vi "车牌字母识别.vi"() -> ()   [LabVIEW 2020]
uses:
  <vilib>/userdefined/High Color/IMAQdx.ctl
  <vilib>/vision/driver/NI_Vision_Acquisition_Software.lvlib
  <vilib>/vision/NI_Vision_Development_Module.lvlib
panel:
  out "Read String":string
  in  "停止":bool
  out "Image":T1(plugin-control)
  in  "Rectangle":T2 {"Rotation" min=-90.0 max=90.0 step=1.0 format="%.2f"; "Left" scale=0.0..1024.0; "Right" scale=0.0..1024.0}
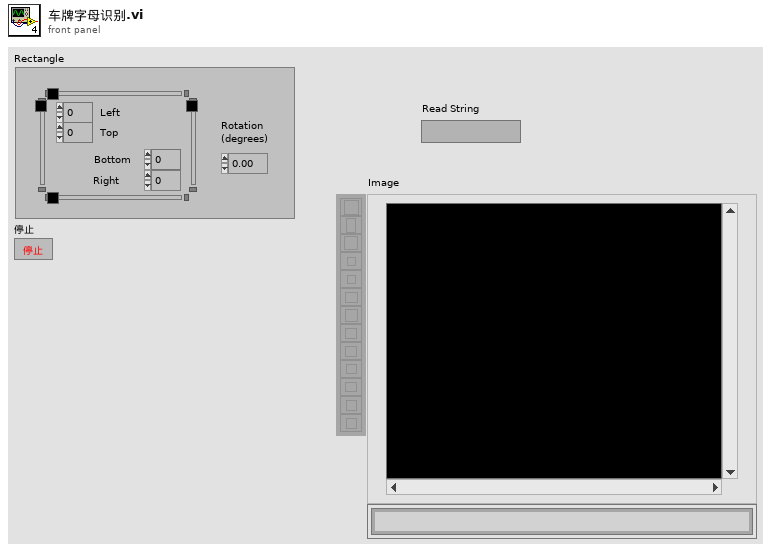
[diagram p1: front panel]
types:
  T1 = typedef "IMAQ Image.ctl" = refnum<image>
  T2 = typedef "IMAQ Rectangle" = cluster{"Left":i32, "Top":i32, "Right":i32, "Bottom":i32, "Rotation":dbl}
  T3 = typedef "IMAQdx.ctl" = refnum<k21>
  T4 = typedef "IMAQ OCR Session.ctl" = refnum<k1>
  T5 = typedef "ROI Descriptor" = cluster{"Global Rectangle":i32[], "Contours":cluster{"ID":enum32{"External", "Internal"}, "Type":u32, "Coordinates":i32[]}[]}
  T6 = cluster{"Global Rectangle":i32[], "Contours":cluster{"ID":enum32{"External", "Internal"}, "Type":u32, "Coordinates":i32[]}[]}
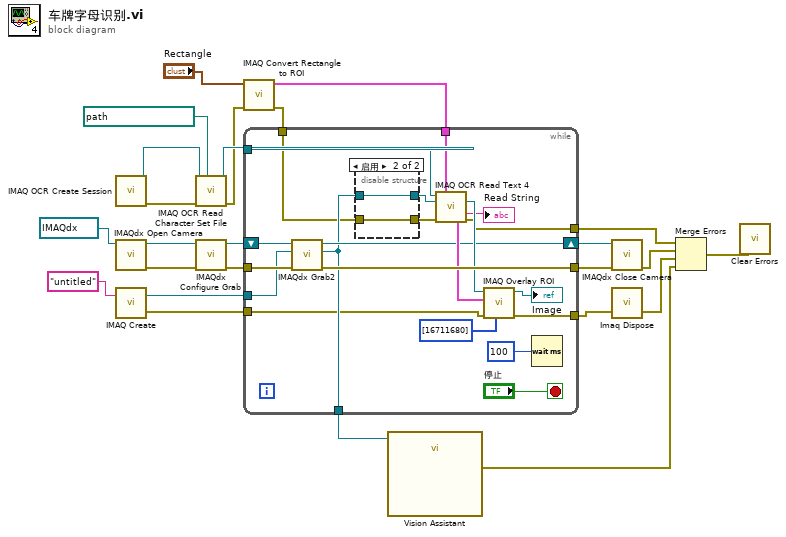
[diagram p0: block diagram]
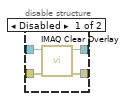
[diagram p2: hidden frame]
diagram:
  n1 = call "IMAQ OCR Create Session"() -> ("error out"=w14:errorcluster, "IMAQ OCR Session"=w15:T4)  [unwired: 10 in]
  n2 = call <vilib>:"IMAQdx Open Camera.vi"("Session In"=T3 "cam1") -> ("error out"=w24:errorcluster, "Session Out"=w25:T3)  [unwired: 9 in]
  n3 = call "IMAQ Create"("Image Name"="untitled") -> ("New Image"=w17:T1, "error out"=w7:errorcluster)  [unwired: 4 in]
  n4 = call "IMAQ OCR Read Character Set File"("File Path"=path "E:/朱晨辉/个人资料/01-计算机编程/00-上位机开发/02-基础知识/09-基于VISION的图像采集V2020/09-车牌字母识别/DetailFile/字母识别.abc", "error in (no error)"=w14, "IMAQ OCR Session"=w15) -> ("error out"=w9:errorcluster, "IMAQ OCR Session (dup)"=w12:T4)  [unwired: 6 in, 1 out]
  n5 = call <vilib>:"IMAQdx Configure Grab.vi"("error in"=w24, "Session In"=w25) -> ("error out"=w22:errorcluster, "Session Out"=w23:T3)  [unwired: 8 in]
  n6 = call "IMAQ Convert Rectangle to ROI"("error in (no error)"=w9, "Rectangle"="Rectangle") -> ("error out"=w8:errorcluster, "ROI Descriptor"=w11:T5)  [unwired: 7 in]
  n7 = while {
    shift-right: [w38] -> w21
    shift-left: w23 -> [w46]
    tunnel: w17 -> [w43]
    tunnel: [w36] -> w16
    tunnel: w12 -> [w37]
    tunnel: w11 -> [w42]
    tunnel: w22 -> [w45]
    tunnel: [w44] -> w20
    tunnel: w8 -> [w30]
    tunnel: [w28] -> w3
    tunnel: w7 -> [w27]
    tunnel: [w26] -> w6
    stop <- "停止" stop-if-true
    n8 = call <vilib>:"IMAQdx Grab2.vi"("error in"=w45, "Image In"=w43, "Session In"=w46) -> ("error out"=w44:errorcluster, "Image Out"=w36:T1, "Session Out"=w38:T3)  [unwired: 5 in, 1 out]
    n9 = disable-structure shown="启用" {
      disable-tunnel: w36 -> [w50 w52]
      disable-tunnel: [w49 w52] -> w35
      disable-tunnel: w30 -> [w48 w51]
      disable-tunnel: [w47 w51] -> w29
      frame Disabled {
        n10 = call "IMAQ Clear Overlay"("error in (no error)"=w48, "Image"=w50) -> ("error out"=w47:errorcluster, "Image Out"=w49:T1)  [unwired: 8 in]
      }
      frame Enabled {
      }
    }
    n11 = call "IMAQ OCR Read Text 4"("IMAQ OCR Session"=w37, "ROI Descriptor"=w42, "Image"=w35, "error in (no error)"=w29) -> ("Image (dup)"=w41:T1, "Read String"=→"Read String":string, "ROI Bounding Characters"=w40:T6, "error out"=w28:errorcluster)  [unwired: 5 in, 3 out]
    n12 = call "IMAQ Overlay ROI"("Colors (Green)"=u32[] [16711680], "error in (no error)"=w27, "ROI Descriptor"=w40, "Image"=w41) -> ("error out"=w26:errorcluster, "Image Out"=→"Image":T1)  [unwired: 6 in]
    n13 = Wait (ms)(milliseconds to wait=u32 100 ("等待时间（毫秒）")) -> ()  [unwired: 1 out]
  }
  n14 = call "Vision Assistant"("Image In"=w16) -> ("error out"=w1:errorcluster)  [unwired: 25 in, 1 out]
  n15 = call <vilib>:"IMAQdx Close Camera.vi"("error in"=w20, "Session In"=w21) -> ("error out"=w4:errorcluster)  [unwired: 9 in]
  n16 = call "Imaq Dispose"("error in (no error)"=w6) -> ("error out"=w5:errorcluster)  [unwired: 5 in]
  n17 = Merge Errors(w3, w4, w5, w1) -> (w2:errorcluster)
  n18 = call <vilib>:"Clear Errors.vi"("error in (no error)"=w2) -> ()  [unwired: 5 in, 2 out]
